vi "Step 3 - Analyze Quantized Lowpass (Lowpass).vi"() -> ()   [LabVIEW 2023]
doc: "Demonstrates how to use the DFD FXP Quantize Coef VI to quantize the coefficients of a floating-point lowpass finite impulse response (FIR) filter and how to use the Filter Analysis Express VI to analyze the characteristics of the quantized filter.\n\nBefore quantizing the filter coefficients of the lowpass filter, this example specifies an appropriate filter structure for the target fixed-point lowpass filter using the DFD Convert Structure VI and scales the filter coefficients using the DFD Scale Filter VI. This example then uses the DFD FXP Quantize Coef VI to quantize the filter coefficients of the lowpass filter and uses the Filter Analysis Express VI to analyze the quantized lowpass filter. This example also uses the DFD FXP Coef Report VI to generate a filter coefficients report, which helps you determine if any underflow or overflow occurs during the quantization."
uses:
  <vilib>/addons/Digital Filter Design/_Objects.llb/DFD Coef Norm Type.ctl
  <vilib>/addons/Digital Filter Design/FXPModel.llb/DFD FXP Quantize Coef (Easy).vi
  <vilib>/addons/Digital Filter Design/NI_DigFilterLicensed.lvlib
panel:
  out "Coefficients Report":string
  out "Magnitude Responses":dynamicdata(graph)
  # "Select Help>>Show Context Help and move the cursor over the VI icon for more information."
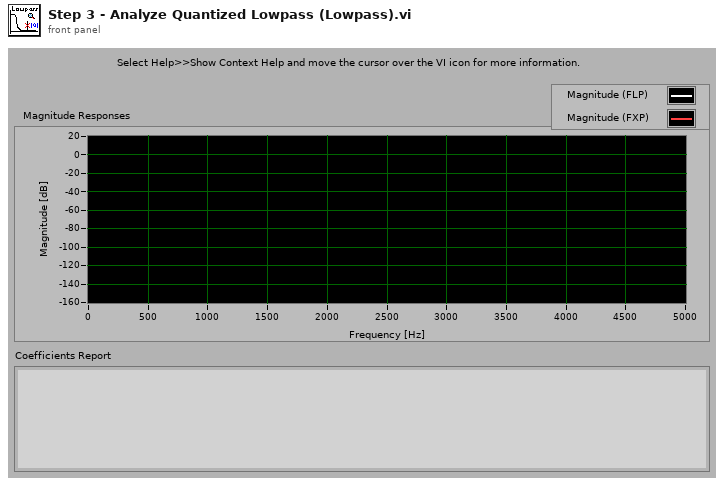
[diagram p1: front panel]
types:
  T1 = typedef "NI_DigFilterLicensed.lvlib/DFD Coef Norm Type.ctl" = enum16{"No Norm", "Time Domain 1-Norm", "Time Domain 2-Norm", "Time Domain Inf-Norm"}
  T2 = typedef "NI_DigFilterLicensed.lvlib/DFD Filter Obj.ctl" = cluster{"mSRate_Fs":dbl, "mSRate_Version":string, "mSRate_Comments":string, "mSRate_OrgCoef":T3, "mSRate_CurCoef":T3, "mSRate_Quantized?":bool, "mSRate_QCoef":T3, "mSRate_QSettings":T5[], "mSRate_Order":i32, "mSRate_Scaling":cluster{"mSRate_ScaleByPowerOf2?":bool, "mSRate_ScaleType":T1}}
  T3 = typedef "NI_DigFilterLicensed.lvlib/DFD Filter Coef.ctl" = cluster{"type":T4, "gain":dbl, "coef a (k)":dbl[], "coef b (v)":dbl[]}
  T4 = typedef "NI_DigFilterLicensed.lvlib/DFD Filter Structure Type Selector.ctl" = enum16{"Undefined", "FIR Direct Form", "FIR Direct Form Transposed", "FIR Symmetric", "FIR Antisymmetric", "IIR Direct Form I", "IIR Direct Form I Transposed", "IIR Direct Form II", "IIR Direct Form II Transposed", "IIR Cascaded Second Order Sections Form I", "IIR Cascaded Second Order Sections Form I Transposed", "IIR Cascaded Second Order Sections Form II", "IIR Cascaded Second Order Sections Form II Transposed", "Lattice Allpass (basic sections)", "Lattice Allpass (one multiplier sections)", "Lattice Allpass (normalized sections)", "Lattice AR (basic sections)", "Lattice AR (one multiplier sections)", "Lattice AR (normalized sections)", "Lattice MA (minimum phase)", "Lattice MA (maximum phase)", "Lattice ARMA (basic sections)", "Lattice ARMA (one multiplier sections)", "Lattice ARMA (normalized sections)"}
  T5 = typedef "NI_DigFilterLicensed.lvlib/dfd_Internal Quantization Settings.ctl" = cluster{"source":T6, "wl":i16, "iwl":i16, "overflow mode":enum16{"Saturation", "Wrap"}, "rounding mode":enum16{"Nearest", "Truncation"}, "signed?":bool}
  T6 = typedef "NI_DigFilterLicensed.lvlib/dfd_Internal Quantization Srcs.ctl" = u16
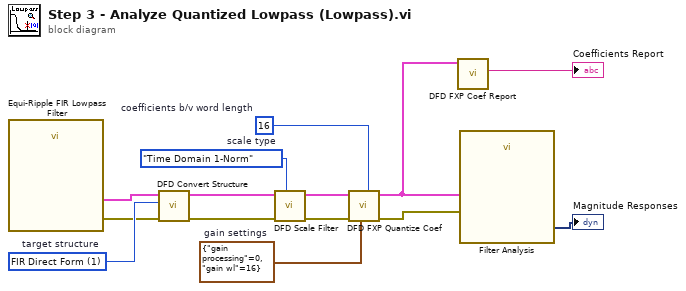
[diagram p0: block diagram]
diagram:
  w6 = u16 1 items=["FIR Direct Form"=1, "FIR Direct Form Transposed"=2, "FIR Symmetric"=3, "FIR Antisymmetric"=4, "IIR Direct Form I"=5, "IIR Direct Form I Transposed"=6, "IIR Direct Form II"=7, "IIR Direct Form II Transposed"=8, "IIR Cascaded Second-Order Sections Form I"=9, "IIR Cascaded Second-Order Sections Form I Transposed"=10, "IIR Cascaded Second-Order Sections Form II"=11, "IIR Cascaded Second-Order Sections Form II Transposed"=12, "Lattice Allpass (basic sections)"=13, "Lattice Allpass (one multiplier sections)"=14, "Lattice Allpass (normalized sections)"=15, "Lattice AR (basic sections)"=16, "Lattice AR (one multiplier sections)"=17, "Lattice AR (normalized sections)"=18, "Lattice MA (minimum phase)"=19, "Lattice MA (maximum phase)"=20, "Lattice ARMA (basic sections)"=21, "Lattice ARMA (one multiplier sections)"=22, "Lattice ARMA (normalized sections)"=23]  # target structure
  w7 = DFD_Coef_Norm_Type."Time Domain 1-Norm"  # scale type
  w13 = i16 16  # coefficients b/v word length
  w12 = cluster{"gain processing":u16, "gain wl":i16} {"gain processing"=0, "gain wl"=16}  # gain settings
  n1 = call "Equi-Ripple FIR Lowpass Filter"() -> ("error out"=w4:errorcluster, "filter out"=w5:T2)  [unwired: 1 in, 9 out]
  n2 = call <vilib>:"DFD Convert Structure.vi"("error in (no error)"=w4, "target structure"=w6, "filter in"=w5) -> ("error out"=w9:errorcluster, "filter out"=w11:T2)  [unwired: 7 out]
  n3 = call <vilib>:"DFD Scale Filter.vi"("scale type"=w7, "error in (no error)"=w9, "filter in"=w11) -> ("error out"=w8:errorcluster, "filter out"=w10:T2)  [unwired: 7 out]
  n4 = call-poly <vilib>:"DFD FXP Quantize Coef.vi"("coefficients b/v word length"=w13, "gain settings"=w12, "error in (no error)"=w8, "filter in"=w10) -> ("error out"=w2:errorcluster, "filter out"=w3:T2)  [unwired: 1 in, 5 out]
  n5 = call <vilib>:"DFD FXP Coef Report.vi"("filter in"=w3) -> ("coefficients report"=→"Coefficients Report":string)  [unwired: 1 in, 9 out]
  n6 = call "Filter Analysis"("error in (no error)"=w2, "filter in"=w3) -> ("magnitude"=→"Magnitude Responses":dynamicdata)  [unwired: 9 out]
